vi "autonSample.vi"(0 "Auton Array":dbl[][](array[numeric]), 5 "LeftEncoder":dbl, 7 "RightEncoder":dbl, 11 "MeasuredHeading":dbl) -> (4 "Left Drive":dbl, 6 "Right Drive":dbl, 8 "Ramp ACT motor":dbl, 10 "Harvester":dbl, 13 "Shooter motor output":dbl, 14 "Turret Rotation":dbl, 15 "Convyeor":dbl)   [LabVIEW 2011]
uses:
  Robot Global Data.vi
panel:
  out "Primitive ID":i16
  out "Tzero":i64
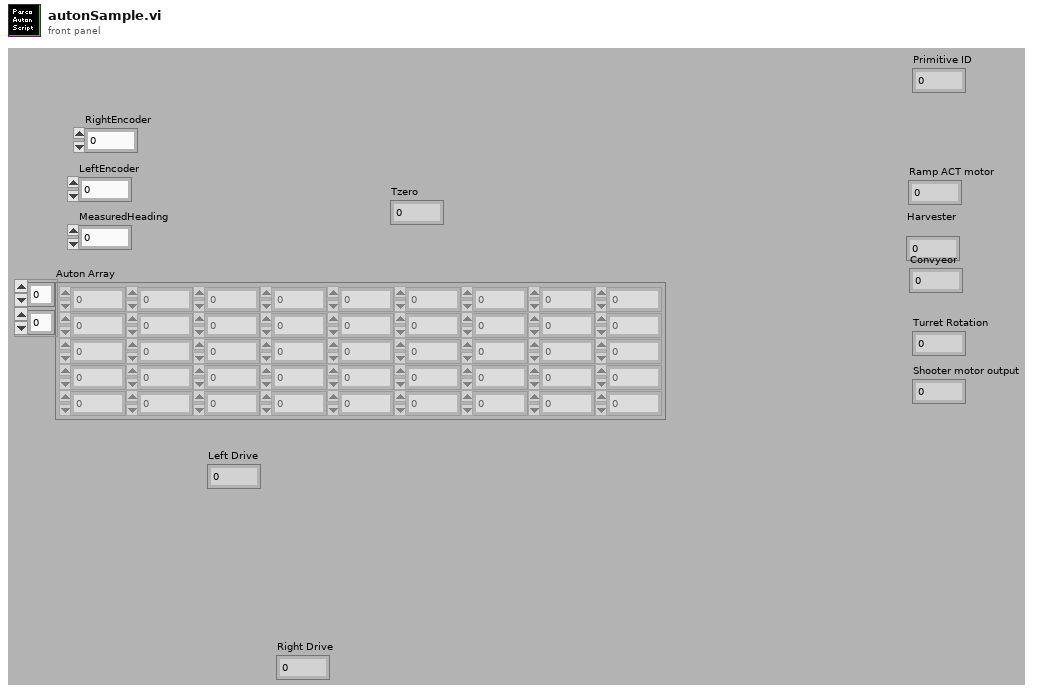
[diagram p1: front panel]
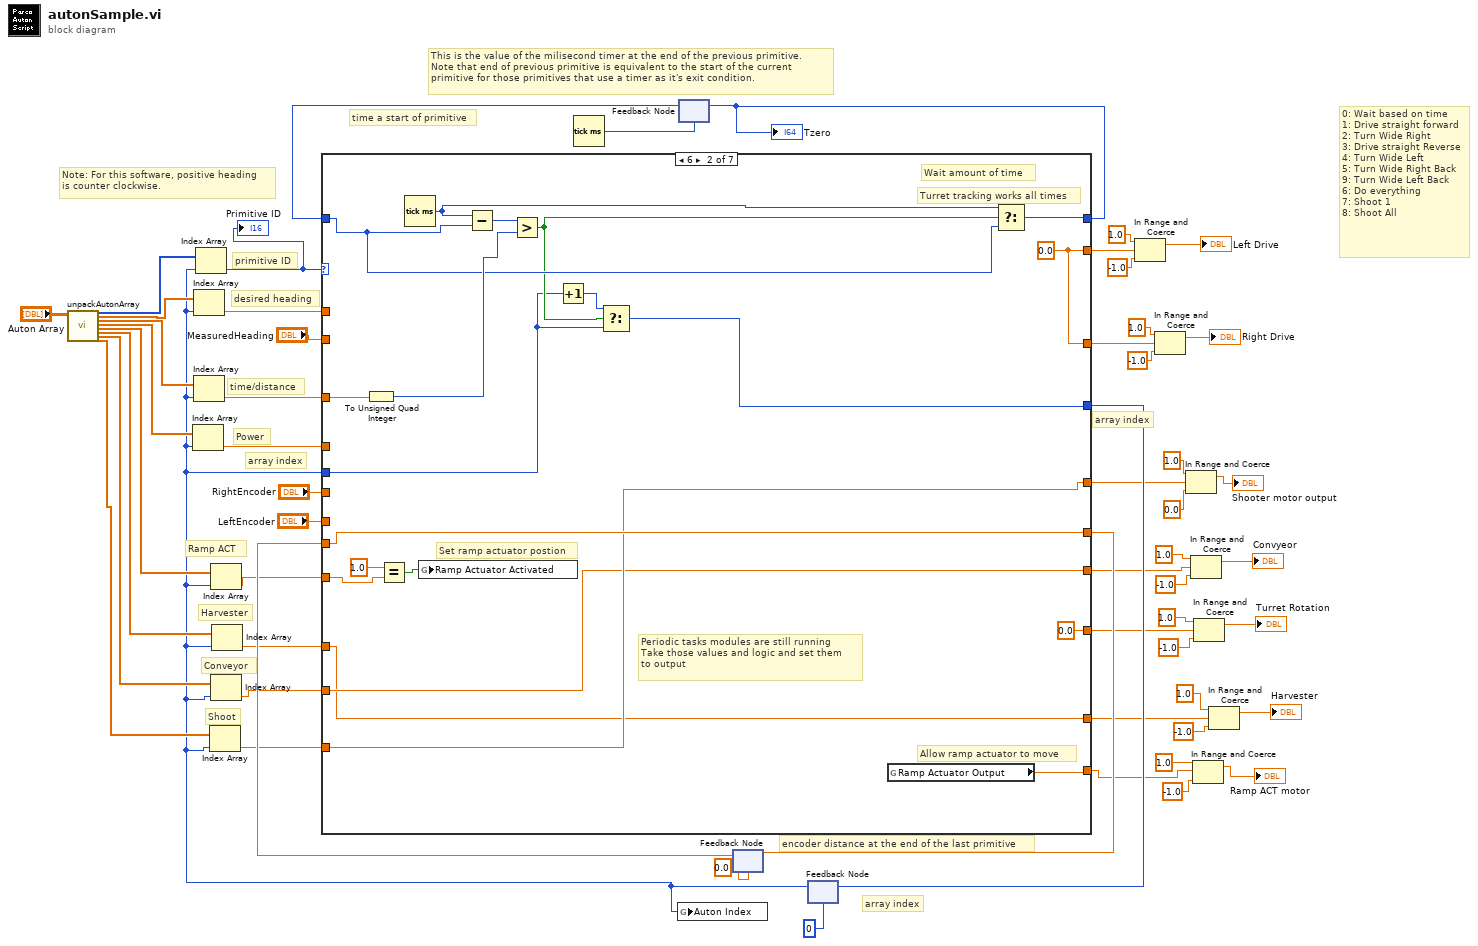
[diagram p0: block diagram]
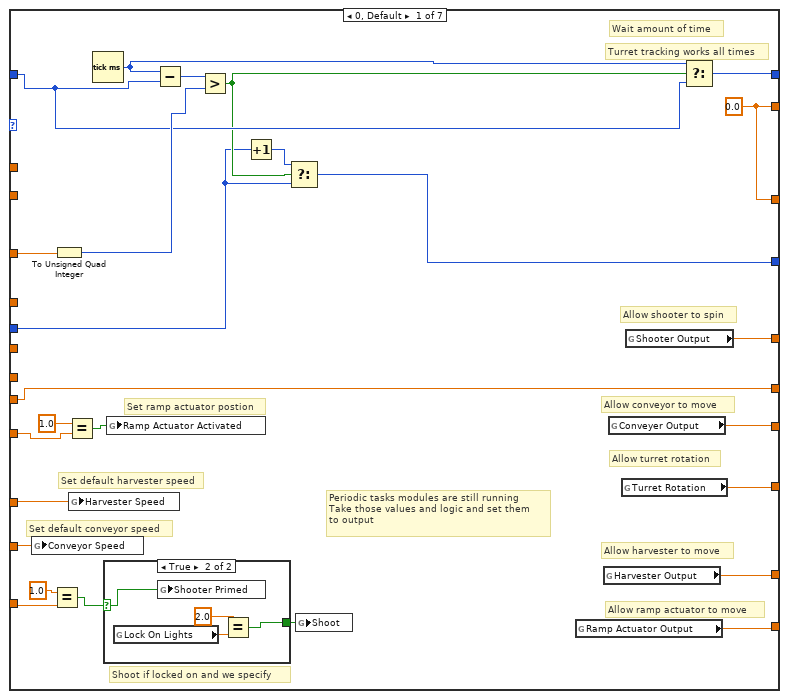
[diagram p2: hidden frame]
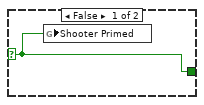
[diagram p3: hidden frame]
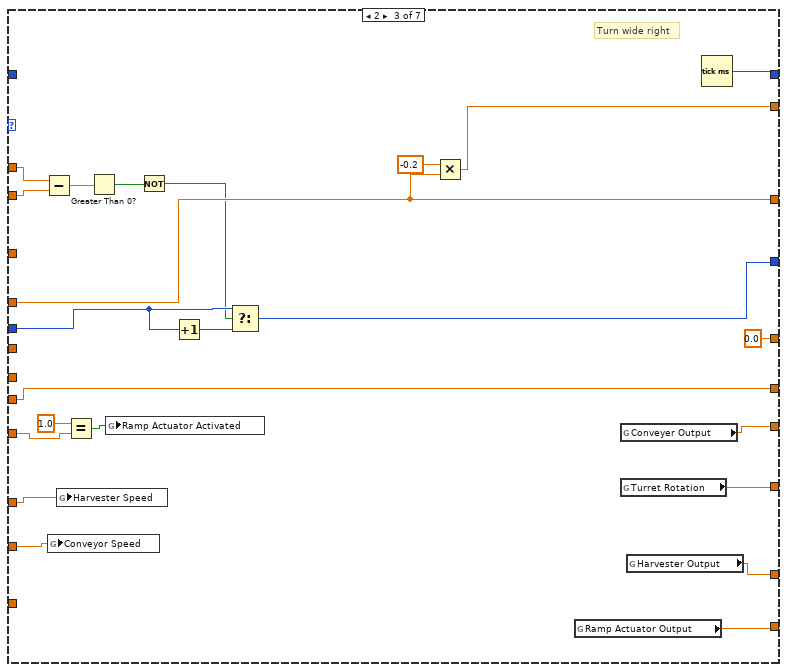
[diagram p4: hidden frame]
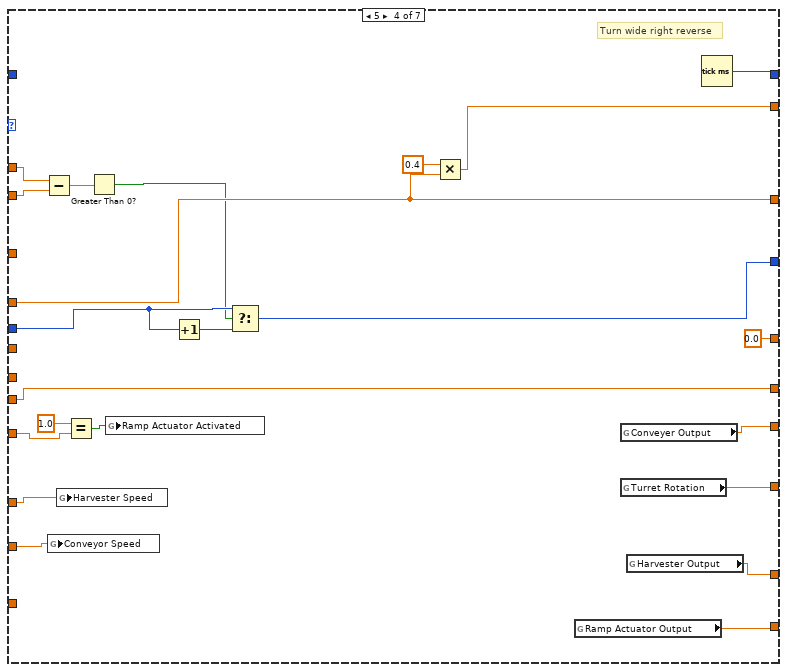
[diagram p5: hidden frame]
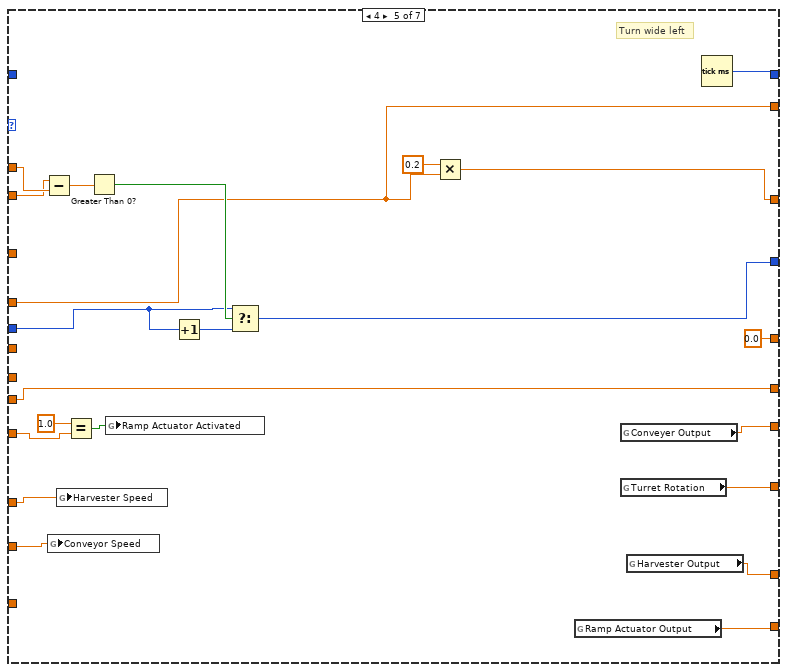
[diagram p6: hidden frame]
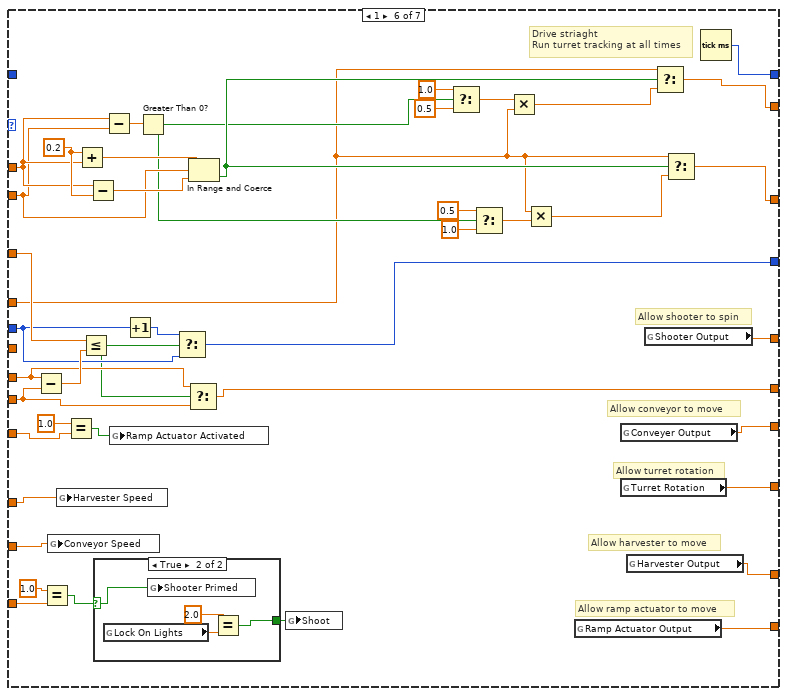
[diagram p7: hidden frame]
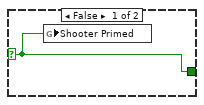
[diagram p8: hidden frame]
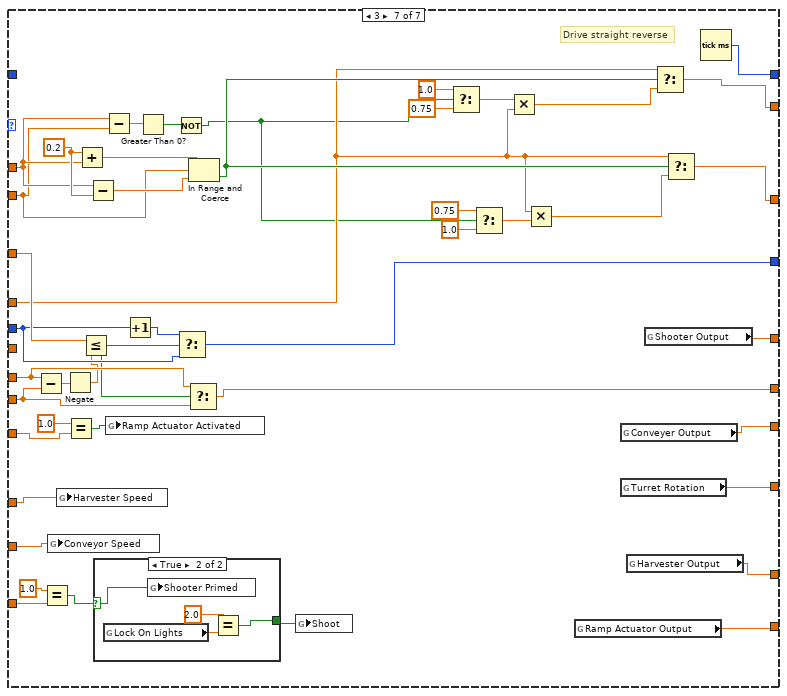
[diagram p9: hidden frame]
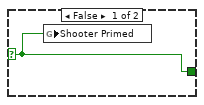
[diagram p10: hidden frame]
diagram:
  # "0: Wait based on time\n1: Drive straight forward\n2: Turn Wide Right\n3: Drive straight Reverse\n4: Turn Wide Left\n5: Turn Wide Right Back\n9: Turn Wide Left Back\n6: Do everything\n7: Shoot 1\n8: Shoot All"
  # "Shoot"
  # "Conveyor"
  # "Harvester"
  # "Ramp ACT"
  # "encoder distance at the end of the last primitive"
  # "Note: For this software, positive heading\nis counter clockwise."
  # "time a start of primitive"
  # "array index"
  # "array index"
  # "This is the value of the milisecond timer at the end of the previous primitive.\nNote that end of previous primitive is equivalent to the start of the current\nprimitive for those primitives that use a timer as it's exit condition."
  # "Power"
  # "array index"
  # "desired heading"
  # "primitive ID"
  # "time/distance"
  n1 = call "unpackAutonArray.vi"("all rows"="Auton Array") -> ("Primitive"=w56:i16[], "Desired Heading"=w16:dbl[], "Time/Distance"=w15:dbl[], "Power"=w14:dbl[], "Ramp Actuator"=w13:dbl[], "Harvester"=w12:dbl[], "Conveyor"=w11:dbl[], "Shoot"=w10:dbl[])  [unwired: 1 in, 18 out]
  n2 = Tick Count (ms)() -> (millisecond timer value=w51:u32)
  n3 = feedback #1(w51) -> (w55:u32)
  n4 = feedback #2(0.0 ("EncoderDistance")) -> (w39:dbl)
  n5 = feedback #3(0) -> (w8:i32)
  n6 = Index Array(array=w14, index=w8) -> (element=w53:dbl)
  n7 = Index Array(array=w16, index=w8) -> (element=w40:dbl)
  n8 = Index Array(array=w15, index=w8) -> (element=w54:dbl)
  n9 = Index Array(array=w56, index=w8) -> (element=w22:i16)
  "Primitive ID" <- w22
  n10 = Index Array(array=w10, index=w8) -> (element=w9:dbl)
  n11 = Index Array(array=w13, index=w8) -> (element=w21:dbl)
  n12 = Index Array(array=w11, index=w8) -> (element=w6:dbl)
  n13 = Index Array(array=w12, index=w8) -> (element=w7:dbl)
  n14 = case shown="6" w22 {
    tunnel: [w75 w100 w111 w133 w159 w201 w252] -> w35
    tunnel: w8 -> [w76 w101 w113 w135 w161 w203 w254]
    tunnel: [w83 w108 w120 w142 w165 w179 w231] -> w41
    tunnel: w55 -> [w80 w105 _ _ _ _ _]
    tunnel: w54 -> [w69 w95 _ _ _ w204 w255]
    tunnel: w40 -> [_ _ w119 w141 w156 w192 w243]
    tunnel: [w74 w99 w115 w137 w158 w178 w230] -> w49
    tunnel: [w74 w99 w117 w139 w157 w177 w229] -> w42
    tunnel: w53 -> [_ _ w117 w139 w158 w181 w233]
    tunnel: "LeftEncoder" -> [_ _ _ _ _ w198 w249]
    tunnel: "MeasuredHeading" -> [_ _ w118 w140 w155 w191 w242]
    tunnel: [w68 w94 w122 w144 w167 w200 w251] -> w36
    tunnel: w39 -> [w68 w94 w122 w144 w167 w199 w250]
    tunnel: [w58 w92 0.0 ("Shooter Output") 0.0 ("Shooter Output") 0.0 ("Shooter Output") w206 w256] -> w31
    tunnel: [w70 0.0 ("Turret Rotation") w128 w150 w172 w216 w265] -> w27
    tunnel: [w66 w90 w124 w146 w169 w210 w260] -> w23
    tunnel: w21 -> [w63 w93 w127 w149 w154 w213 w228]
    tunnel: [w71 w96 w129 w151 w173 w217 w266] -> w20
    tunnel: w9 -> [w59 w92 _ _ _ w214 w263]
    tunnel: w7 -> [w64 w90 w126 w148 w171 w212 w262]
    tunnel: w6 -> [w65 w91 w125 w147 w170 w211 w261]
    tunnel: [w67 w91 w123 w145 w168 w209 w259] -> w2
    tunnel: "RightEncoder" -> [_ _ _ _ _ _ _]
    frame 0, Default {
      w74 = 0.0 ("Numeric")
      # "Periodic tasks modules are still running\nTake those values and logic and set them \nto output"
      # "Set ramp actuator postion"
      # "Set default harvester speed"
      # "Set default conveyor speed"
      # "Shoot if locked on and we specify"
      # "Allow ramp actuator to move"
      # "Allow harvester to move"
      # "Turret tracking works all times"
      # "Allow turret rotation"
      # "Allow conveyor to move"
      # "Allow shooter to spin"
      # "Wait amount of time"
      n15 = global write "Robot Global Data.vi" "Conveyor Speed"(w65) -> ()
      n16 = Equal?(x=1.0, y=w59) -> (x = y?=w61:bool)
      n17 = To Unsigned Quad Integer(1:w69) -> (0:w81:u64)
      n18 = Equal?(x=1.0, y=w63) -> (x = y?=w72:bool)
      n19 = global write "Robot Global Data.vi" "Harvester Speed"(w64) -> ()
      n20 = Tick Count (ms)() -> (millisecond timer value=w79:u32)
      n21 = case shown="True" w61 {
        selector: w61 -> [w84 w88]
        tunnel: [w84 w85] -> w60
        frame False {
          n22 = global write "Robot Global Data.vi" "Shooter Primed"(w84) -> ()
        }
        frame True {
          n23 = global read "Robot Global Data.vi" "Lock On Lights"() -> (w86:dbl)
          n24 = global write "Robot Global Data.vi" "Shooter Primed"(w88) -> ()
          n25 = Equal?(x=2.0, y=w86) -> (x = y?=w85:bool)
        }
      }
      n26 = global write "Robot Global Data.vi" "Ramp Actuator Activated"(w72) -> ()
      n27 = Subtract(x=w79, y=w80) -> (x-y=w82:u32)
      n28 = Greater?(x=w82, y=w81) -> (0:w78:bool)
      n29 = Increment(x=w76) -> (x+1=w77:i32)
      n30 = Select(t=w77, s=w78, f=w76) -> (s? t:f=w75:i32)
      n31 = global write "Robot Global Data.vi" "Shoot"(w60) -> ()
      n32 = global read "Robot Global Data.vi" "Ramp Actuator Output"() -> (w71:dbl)
      n33 = global read "Robot Global Data.vi" "Harvester Output"() -> (w66:dbl)
      n34 = global read "Robot Global Data.vi" "Conveyer Output"() -> (w67:dbl)
      n35 = global read "Robot Global Data.vi" "Turret Rotation"() -> (w70:dbl)
      n36 = global read "Robot Global Data.vi" "Shooter Output"() -> (w58:dbl)
      n37 = Select(t=w79, s=w78, f=w80) -> (s? t:f=w83:u32)
    }
    frame 6 {
      w99 = 0.0 ("Numeric")
      # "Periodic tasks modules are still running\nTake those values and logic and set them \nto output"
      # "Set ramp actuator postion"
      # "Allow ramp actuator to move"
      # "Turret tracking works all times"
      # "Wait amount of time"
      n38 = To Unsigned Quad Integer(1:w95) -> (0:w106:u64)
      n39 = Equal?(x=1.0, y=w93) -> (x = y?=w97:bool)
      n40 = Tick Count (ms)() -> (millisecond timer value=w104:u32)
      n41 = global write "Robot Global Data.vi" "Ramp Actuator Activated"(w97) -> ()
      n42 = Subtract(x=w104, y=w105) -> (x-y=w107:u32)
      n43 = Greater?(x=w107, y=w106) -> (0:w103:bool)
      n44 = Increment(x=w101) -> (x+1=w102:i32)
      n45 = Select(t=w102, s=w103, f=w101) -> (s? t:f=w100:i32)
      n46 = global read "Robot Global Data.vi" "Ramp Actuator Output"() -> (w96:dbl)
      n47 = Select(t=w104, s=w103, f=w105) -> (s? t:f=w108:u32)
    }
    frame 2 {
      # "Turn wide right"
      n48 = Subtract(x=w119, y=w118) -> (x-y=w114:dbl)
      n49 = global write "Robot Global Data.vi" "Conveyor Speed"(w125) -> ()
      n50 = global write "Robot Global Data.vi" "Harvester Speed"(w126) -> ()
      n51 = Equal?(x=1.0, y=w127) -> (x = y?=w130:bool)
      n52 = Greater Than 0?(x=w114) -> (x > 0?=w110:bool)
      n53 = global write "Robot Global Data.vi" "Ramp Actuator Activated"(w130) -> ()
      n54 = Not(x=w110) -> (.not. x?=w109:bool)
      n55 = Increment(x=w113) -> (x+1=w112:i32)
      n56 = Select(t=w113, s=w109, f=w112) -> (s? t:f=w111:i32)
      n57 = Multiply(x=-0.2, y=w117) -> (x*y=w115:dbl)
      n58 = global read "Robot Global Data.vi" "Ramp Actuator Output"() -> (w129:dbl)
      n59 = global read "Robot Global Data.vi" "Conveyer Output"() -> (w123:dbl)
      n60 = global read "Robot Global Data.vi" "Turret Rotation"() -> (w128:dbl)
      n61 = global read "Robot Global Data.vi" "Harvester Output"() -> (w124:dbl)
      n62 = Tick Count (ms)() -> (millisecond timer value=w120:u32)
    }
    frame 5 {
      # "Turn wide right reverse"
      n63 = Subtract(x=w141, y=w140) -> (x-y=w136:dbl)
      n64 = global write "Robot Global Data.vi" "Conveyor Speed"(w147) -> ()
      n65 = global write "Robot Global Data.vi" "Harvester Speed"(w148) -> ()
      n66 = Equal?(x=1.0, y=w149) -> (x = y?=w152:bool)
      n67 = Greater Than 0?(x=w136) -> (x > 0?=w132:bool)
      n68 = global write "Robot Global Data.vi" "Ramp Actuator Activated"(w152) -> ()
      n69 = Increment(x=w135) -> (x+1=w134:i32)
      n70 = Select(t=w135, s=w132, f=w134) -> (s? t:f=w133:i32)
      n71 = Multiply(x=0.4, y=w139) -> (x*y=w137:dbl)
      n72 = global read "Robot Global Data.vi" "Ramp Actuator Output"() -> (w151:dbl)
      n73 = global read "Robot Global Data.vi" "Conveyer Output"() -> (w145:dbl)
      n74 = global read "Robot Global Data.vi" "Turret Rotation"() -> (w150:dbl)
      n75 = global read "Robot Global Data.vi" "Harvester Output"() -> (w146:dbl)
      n76 = Tick Count (ms)() -> (millisecond timer value=w142:u32)
    }
    frame 4 {
      # "Turn wide left"
      n77 = Subtract(x=w155, y=w156) -> (x-y=w163:dbl)
      n78 = global write "Robot Global Data.vi" "Conveyor Speed"(w170) -> ()
      n79 = global write "Robot Global Data.vi" "Harvester Speed"(w171) -> ()
      n80 = Equal?(x=1.0, y=w154) -> (x = y?=w174:bool)
      n81 = Greater Than 0?(x=w163) -> (x > 0?=w162:bool)
      n82 = global write "Robot Global Data.vi" "Ramp Actuator Activated"(w174) -> ()
      n83 = Increment(x=w161) -> (x+1=w160:i32)
      n84 = Select(t=w161, s=w162, f=w160) -> (s? t:f=w159:i32)
      n85 = Multiply(x=0.2, y=w158) -> (x*y=w157:dbl)
      n86 = global read "Robot Global Data.vi" "Ramp Actuator Output"() -> (w173:dbl)
      n87 = global read "Robot Global Data.vi" "Conveyer Output"() -> (w168:dbl)
      n88 = global read "Robot Global Data.vi" "Turret Rotation"() -> (w172:dbl)
      n89 = global read "Robot Global Data.vi" "Harvester Output"() -> (w169:dbl)
      n90 = Tick Count (ms)() -> (millisecond timer value=w165:u32)
    }
    frame 1 {
      w196 = 0.2 ("x")
      # "Allow ramp actuator to move"
      # "Allow harvester to move"
      # "Allow turret rotation"
      # "Allow conveyor to move"
      # "Allow shooter to spin"
      # "Drive striaght\nRun turret tracking at all times"
      n91 = Subtract(x=w198, y=w199) -> (x-y=w205:dbl)
      n92 = Equal?(x=1.0, y=w214) -> (x = y?=w208:bool)
      n93 = global write "Robot Global Data.vi" "Conveyor Speed"(w211) -> ()
      n94 = global write "Robot Global Data.vi" "Harvester Speed"(w212) -> ()
      n95 = Equal?(x=1.0, y=w213) -> (x = y?=w176:bool)
      n96 = Add(x=w196, y=w192) -> (x+y=w194:dbl)
      n97 = Less Or Equal?(x=w204, y=w205) -> (x <= y?=w197:bool)
      n98 = Subtract(x=w192, y=w196) -> (x-y=w195:dbl)
      n99 = case shown="True" w208 {
        selector: w208 -> [w219 w223]
        tunnel: [w219 w220] -> w207
        frame False {
          n100 = global write "Robot Global Data.vi" "Shooter Primed"(w219) -> ()
        }
        frame True {
          n101 = global read "Robot Global Data.vi" "Lock On Lights"() -> (w221:dbl)
          n102 = global write "Robot Global Data.vi" "Shooter Primed"(w223) -> ()
          n103 = Equal?(x=2.0, y=w221) -> (x = y?=w220:bool)
        }
      }
      n104 = Subtract(x=w192, y=w191) -> (x-y=w190:dbl)
      n105 = global write "Robot Global Data.vi" "Ramp Actuator Activated"(w176) -> ()
      n106 = Increment(x=w203) -> (x+1=w202:i32)
      n107 = Greater Than 0?(x=w190) -> (x > 0?=w189:bool)
      n108 = Select(t=w202, s=w197, f=w203) -> (s? t:f=w201:i32)
      n109 = Select(t=w198, s=w197, f=w199) -> (s? t:f=w200:dbl)
      n110 = In Range and Coerce(upper limit=w194, x=w191, lower limit=w195) -> (In Range?=w193:bool)  [unwired: 1 out]
      n111 = global write "Robot Global Data.vi" "Shoot"(w207) -> ()
      n112 = Select(t=1.0, s=w189, f=0.5) -> (s? t:f=w182:dbl)
      n113 = Select(t=0.5, s=w189, f=1.0) -> (s? t:f=w184:dbl)
      n114 = Multiply(x=w182, y=w181) -> (x*y=w180:dbl)
      n115 = Multiply(x=w181, y=w184) -> (x*y=w183:dbl)
      n116 = global read "Robot Global Data.vi" "Ramp Actuator Output"() -> (w217:dbl)
      n117 = global read "Robot Global Data.vi" "Conveyer Output"() -> (w209:dbl)
      n118 = global read "Robot Global Data.vi" "Turret Rotation"() -> (w216:dbl)
      n119 = global read "Robot Global Data.vi" "Harvester Output"() -> (w210:dbl)
      n120 = global read "Robot Global Data.vi" "Shooter Output"() -> (w206:dbl)
      n121 = Select(t=w181, s=w193, f=w180) -> (s? t:f=w178:dbl)
      n122 = Select(t=w181, s=w193, f=w183) -> (s? t:f=w177:dbl)
      n123 = Tick Count (ms)() -> (millisecond timer value=w179:u32)
    }
    frame 3 {
      w247 = 0.2 ("x")
      # "Drive straight reverse"
      n124 = Subtract(x=w249, y=w250) -> (x-y=w227:dbl)
      n125 = Equal?(x=1.0, y=w263) -> (x = y?=w258:bool)
      n126 = global write "Robot Global Data.vi" "Conveyor Speed"(w261) -> ()
      n127 = global write "Robot Global Data.vi" "Harvester Speed"(w262) -> ()
      n128 = Negate(x=w227) -> (-x=w226:dbl)
      n129 = Equal?(x=1.0, y=w228) -> (x = y?=w267:bool)
      n130 = Add(x=w247, y=w243) -> (x+y=w245:dbl)
      n131 = Less Or Equal?(x=w255, y=w226) -> (x <= y?=w248:bool)
      n132 = Subtract(x=w243, y=w247) -> (x-y=w246:dbl)
      n133 = case shown="True" w258 {
        selector: w258 -> [w269 w273]
        tunnel: [w269 w270] -> w257
        frame False {
          n134 = global write "Robot Global Data.vi" "Shooter Primed"(w269) -> ()
        }
        frame True {
          n135 = global read "Robot Global Data.vi" "Lock On Lights"() -> (w271:dbl)
          n136 = global write "Robot Global Data.vi" "Shooter Primed"(w273) -> ()
          n137 = Equal?(x=2.0, y=w271) -> (x = y?=w270:bool)
        }
      }
      n138 = Subtract(x=w243, y=w242) -> (x-y=w241:dbl)
      n139 = global write "Robot Global Data.vi" "Ramp Actuator Activated"(w267) -> ()
      n140 = Increment(x=w254) -> (x+1=w253:i32)
      n141 = Greater Than 0?(x=w241) -> (x > 0?=w225:bool)
      n142 = Not(x=w225) -> (.not. x?=w224:bool)
      n143 = Select(t=w253, s=w248, f=w254) -> (s? t:f=w252:i32)
      n144 = Select(t=w249, s=w248, f=w250) -> (s? t:f=w251:dbl)
      n145 = In Range and Coerce(upper limit=w245, x=w242, lower limit=w246) -> (In Range?=w244:bool)  [unwired: 1 out]
      n146 = global write "Robot Global Data.vi" "Shoot"(w257) -> ()
      n147 = Select(t=1.0, s=w224, f=0.75) -> (s? t:f=w234:dbl)
      n148 = Select(t=0.75, s=w224, f=1.0) -> (s? t:f=w236:dbl)
      n149 = Multiply(x=w234, y=w233) -> (x*y=w232:dbl)
      n150 = Multiply(x=w233, y=w236) -> (x*y=w235:dbl)
      n151 = global read "Robot Global Data.vi" "Ramp Actuator Output"() -> (w266:dbl)
      n152 = global read "Robot Global Data.vi" "Conveyer Output"() -> (w259:dbl)
      n153 = global read "Robot Global Data.vi" "Turret Rotation"() -> (w265:dbl)
      n154 = global read "Robot Global Data.vi" "Harvester Output"() -> (w260:dbl)
      n155 = global read "Robot Global Data.vi" "Shooter Output"() -> (w256:dbl)
      n156 = Select(t=w233, s=w244, f=w232) -> (s? t:f=w230:dbl)
      n157 = Select(t=w233, s=w244, f=w235) -> (s? t:f=w229:dbl)
      n158 = Tick Count (ms)() -> (millisecond timer value=w231:u32)
    }
  }
  "Tzero" <- w41
  n159 = global write "Robot Global Data.vi" "Auton Index"(w8) -> ()
  n160 = feedback-in #1(w41) -> ()
  n161 = feedback-in #2(w36) -> ()
  n162 = feedback-in #3(w35) -> ()
  n163 = In Range and Coerce(upper limit=1.0, x=w49, lower limit=-1.0) -> (coerced(x)=→"Left Drive":dbl)  [unwired: 1 out]
  n164 = In Range and Coerce(upper limit=1.0, x=w42, lower limit=-1.0) -> (coerced(x)=→"Right Drive":dbl)  [unwired: 1 out]
  n165 = In Range and Coerce(upper limit=1.0, x=w31, lower limit=0.0) -> (coerced(x)=→"Shooter motor output":dbl)  [unwired: 1 out]
  n166 = In Range and Coerce(upper limit=1.0, x=w2, lower limit=-1.0) -> (coerced(x)=→"Convyeor":dbl)  [unwired: 1 out]
  n167 = In Range and Coerce(upper limit=1.0, x=w20, lower limit=-1.0) -> (coerced(x)=→"Ramp ACT motor":dbl)  [unwired: 1 out]
  n168 = In Range and Coerce(upper limit=1.0, x=w27, lower limit=-1.0) -> (coerced(x)=→"Turret Rotation":dbl)  [unwired: 1 out]
  n169 = In Range and Coerce(upper limit=1.0, x=w23, lower limit=-1.0) -> (coerced(x)=→"Harvester":dbl)  [unwired: 1 out]
